vi "Update List.vi"(5 "ZeroOffset":i32, 7 "Data":T1[](array[typedef]) {"Direction" items=["Tx", "Rx"]; "CANType" items=["CAN", "CANFD", "CANFD加速"]}, 9 "Pause":bool, 10 "Scroll":refnum<vi>, 11 "List":refnum<vi>) -> ()   [LabVIEW 2011, in "CAN FD.lvlib"]
uses:
  CAN FD.lvlib
  Typedef/CAN Data.ctl
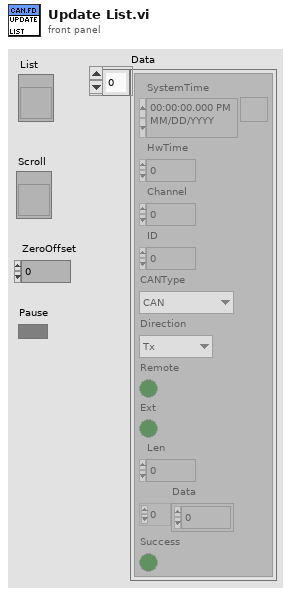
[diagram p1: front panel]
types:
  T1 = typedef "CAN FD.lvlib/CAN Data.ctl" = cluster{"SystemTime":timestamp, "HwTime":dbl, "Channel":u8, "ID":u32, "CANType":i16, "Direction":i16, "Remote":bool, "Ext":bool, "Len":u8, "Data":u8[], "Success":bool}
  T2 = typedef "LVRowAndColumnUnsignedTypeDef.ctl" = cluster{"Row":u32, "Column":u32}
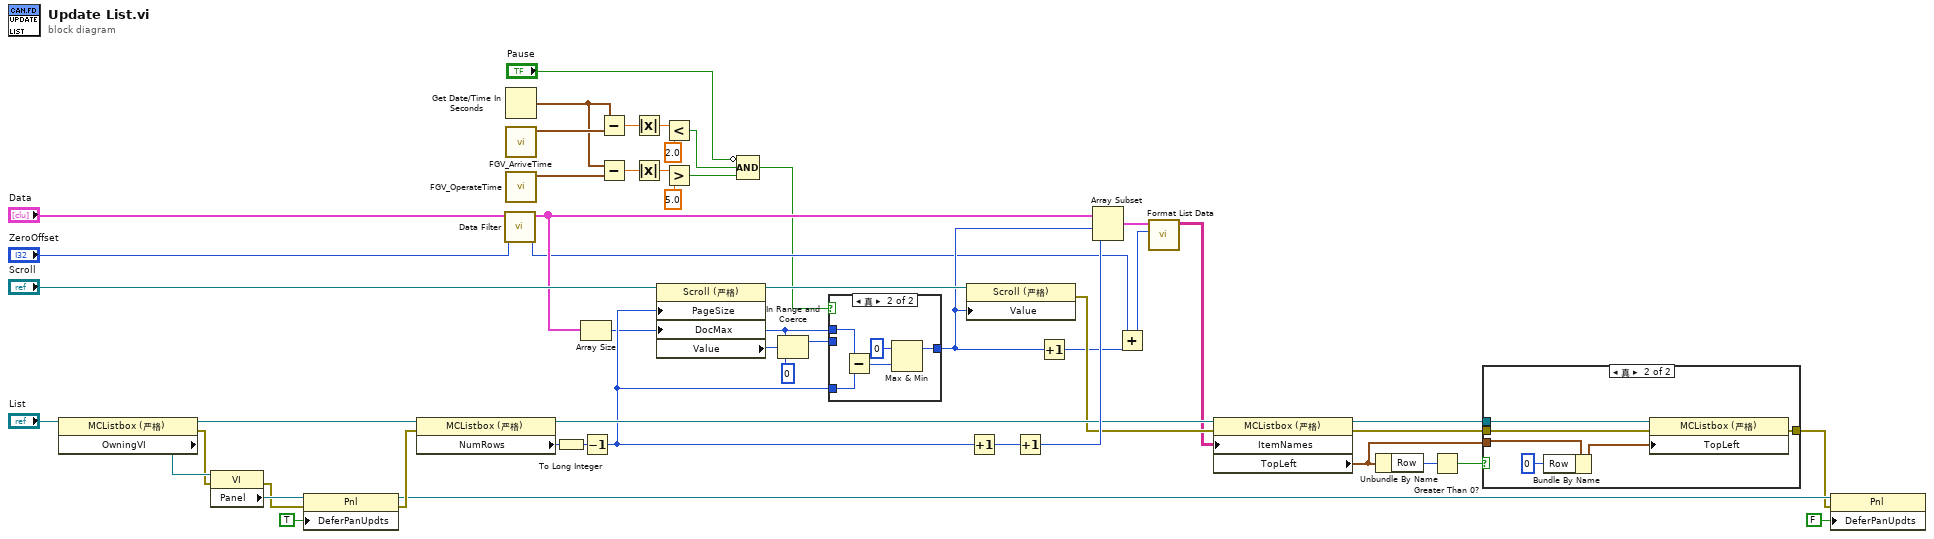
[diagram p0: block diagram]
diagram:
  n1 = property class="MCListbox (严格)"(reference="List") -> (reference out=w47:refnum<vi>, error out=w46:errorcluster, "OwningVI"=w48:refnum<vi>)  [unwired: 1 in]
  n2 = property class="VI"(reference=w48, error in=w46) -> (error out=w45:errorcluster, "Panel"=w50:refnum<vi>)  [unwired: 1 out]
  n3 = property class="Pnl"(reference=w50, error in=w45, "DeferPanUpdts"=TRUE ("延迟前面板更新")) -> (reference out=w34:refnum<vi>, error out=w44:errorcluster)
  n4 = property class="MCListbox (严格)"(reference=w47, error in=w44) -> (reference out=w31:refnum<vi>, "NumRows"=w36:u32)  [unwired: 1 out]
  n5 = call "Data Filter.vi"("ZeroOffset"="ZeroOffset", "Data"="Data") -> ("ZeroOffset out"=w15:i32, "Data out"=w37:T1[])  [unwired: 8 in]
  n6 = Get Date/Time In Seconds() -> (seconds since 1Jan1904=w12:timestamp)
  n7 = call "FGV_ArriveTime.vi"() -> ("ArriveTime out"=w13:timestamp)  [unwired: 10 in, 1 out]
  n8 = call "FGV_OperateTime.vi"() -> ("OperateTime out"=w11:timestamp)  [unwired: 10 in, 1 out]
  n9 = To Long Integer(number=w36) -> (32bit integer=w28:i32)
  n10 = Array Size(array=w37) -> (size(s)=w26:i32)
  n11 = Decrement(x=w28) -> (x-1=w29:i32)
  n12 = Subtract(x=w12, y=w13) -> (x-y=w10:dbl)
  n13 = Subtract(x=w12, y=w11) -> (x-y=w9:dbl)
  n14 = Absolute Value(x=w10) -> (abs(x)=w8:dbl)
  n15 = Absolute Value(x=w9) -> (abs(x)=w5:dbl)
  n16 = property class="Scroll (严格)"(reference="Scroll", "PageSize"=w29, "DocMax"=w26) -> (reference out=w38:refnum<vi>, "Value"=w42:i32)  [unwired: 1 in, 1 out]
  n17 = Less?(x=w8, y=2.0) -> (x < y?=w3:bool)
  n18 = Greater?(x=w5, y=5.0) -> (0:w4:bool)
  n19 = Compound Arithmetic op=AND(invert "Pause", w3, w4) -> (w2:bool)
  n20 = In Range and Coerce(upper limit=w26, x=w42, lower limit=0 ("下限")) -> (coerced(x)=w39:i32)  [unwired: 1 out]
  n21 = case shown="真" w2 {
    tunnel: w26 -> [_ w57]
    tunnel: w29 -> [_ w56]
    tunnel: [w52 w53] -> w32
    tunnel: w39 -> [w52 _]
    frame False {
    }
    frame True {
      n22 = Subtract(x=w57, y=w56) -> (x-y=w55:i32)
      n23 = Max & Min(x=0, y=w55) -> (max(x,y)=w53:i32)  [unwired: 1 out]
    }
  }
  n24 = property class="Scroll (严格)"(reference=w38, "Value"=w32) -> (error out=w30:errorcluster)  [unwired: 1 in, 1 out]
  n25 = Increment(x=w29) -> (x+1=w27:i32)
  n26 = Increment(x=w27) -> (x+1=w35:i32)
  n27 = Increment(x=w32) -> (x+1=w16:i32)
  n28 = Array Subset(array=w37, index=w32, length=w35) -> (w25:T1[])
  n29 = Add(x=w15, y=w16) -> (x+y=w14:i32)
  n30 = call "Format List Data.vi"("#Offset"=w14, "Data"=w25) -> ("List Data"=w24:string[][])  [unwired: 9 in]
  n31 = property class="MCListbox (严格)"(reference=w31, error in=w30, "ItemNames"=w24) -> (reference out=w19:refnum<vi>, error out=w20:errorcluster, "TopLeft"=w18:T2)
  n32 = Unbundle By Name(w18) -> ("Row"=w23:u32)
  n33 = Greater Than 0?(x=w23) -> (x > 0?=w22:bool)
  n34 = case shown="真" w22 {
    tunnel: [w58 w63] -> w21
    tunnel: w20 -> [w58 w62]
    tunnel: w19 -> [_ w64]
    tunnel: w18 -> [_ w61]
    frame False {
    }
    frame True {
      n35 = Bundle By Name(cluster=w61, "Row"=u32 0) -> (w59:T2)
      n36 = property class="MCListbox (严格)"(reference=w64, error in=w62, "TopLeft"=w59) -> (error out=w63:errorcluster)  [unwired: 1 out]
    }
  }
  n37 = property class="Pnl"(reference=w34, error in=w21, "DeferPanUpdts"=FALSE ("延迟前面板更新")) -> ()  [unwired: 2 out]
